vi "ADC Data capture and Process_new.vi"(0 "ADC Output Read Method":T2(ring)=enum."Read .dat file", 1 "Select the Tab to project":T1(ring)=enum."ADC Sine", 2 "ADC Input":enum16{"Sine Wave", "Ramp / Triangle"}(ring), 3 "No.of samples(SNR)":i32=4096, 4 "Resolution":i32=12, 5 "active edge":i32(ring)=10280, 6 "Inputs for Dyanmic para":T9={"Fundamental Frequency"=100000.0, "Sampling Frequncy"=3999610.0, "No of Harmonics"=9, "Window"=enum."7 Term B-Harris", "Blackman (fundamental power) bins)"=1.0}, 7 "Samples per Channel":i32=4096 caption="No.of Samples(capture)", 8 "Oversampling":bool, 9 "Oversampling ratio":i32, 10 "Drop LSB":bool, 11 "Save data":T15, 12 "Waveform":i64[](array[numeric]), 13 "Path to Read":path=path "C/Users/a0230227/Desktop/save.dat", 14 "Start & Stop Bit":cluster{"Start":i32, "Stop":i32}={"Start"=40, "Stop"=4055}, 15 "length":i32=4096, 17 "Set_Freq":dbl=100017.0, 24 "path to save":T14={"Path to Save plot"=path "D/Tenor_176P/DYN_PAR_C004/DAT/D001_TEMPP30C_VDD1.2_VDDA3.3_16B_SE_ADCA__vicA_aggX_PLT_CAP_200821_1740_33.jpg", "Path to Raw Data plot"=path "D/Tenor_176P/DYN_PAR_C004/DAT/D001_TEMPP30C_VDD1.2_VDDA3.3_16B_SE_ADCA__vicA_aggX_RAW_DAT_200821_1740_33.csv"}) -> (18 "Min Max":T4, 19 "detected Throughput":dbl, 20 "output cluster":T7, 21 "Dynamic Parameters":T8, 22 "max code":ext, 23 "min code":ext, 25 "Valid Capture":bool)   [LabVIEW 2019] (continued)
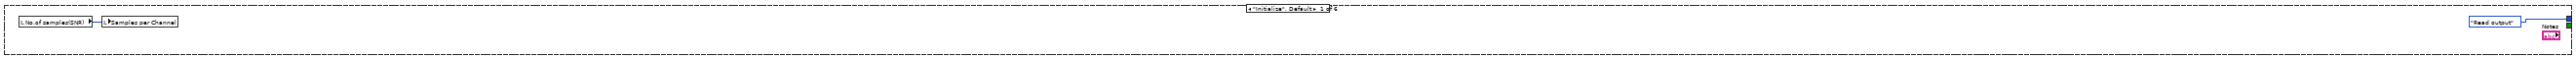
[diagram p2: hidden frame]
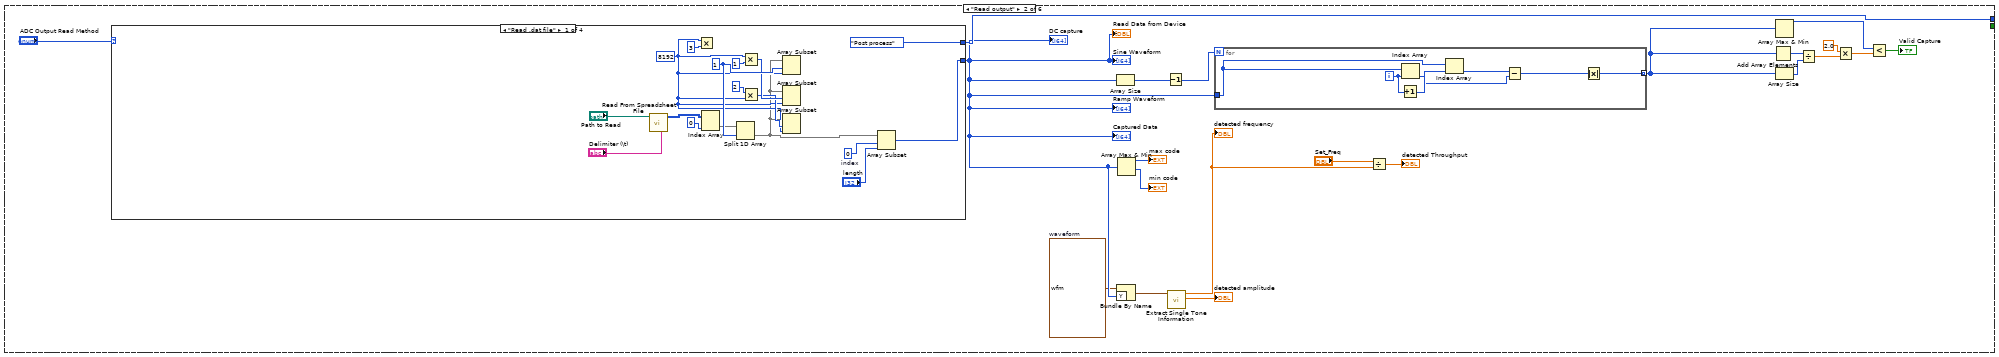
[diagram p3: hidden frame]
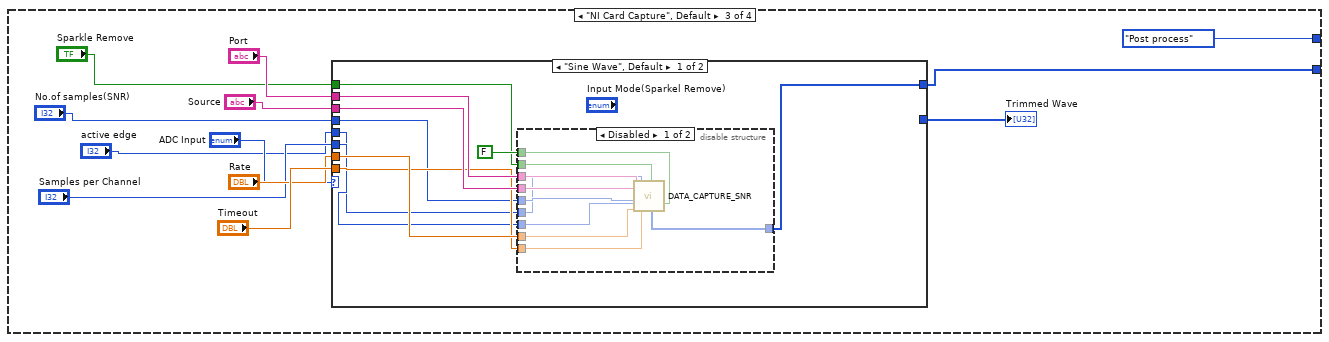
[diagram p5: hidden frame]
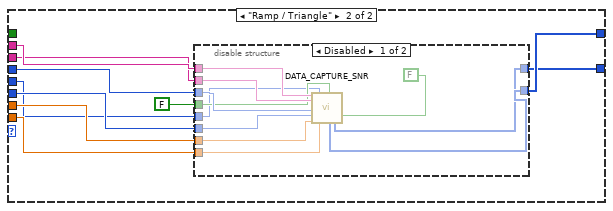
[diagram p7: hidden frame]
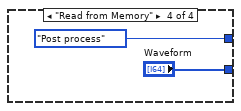
[diagram p9: hidden frame]
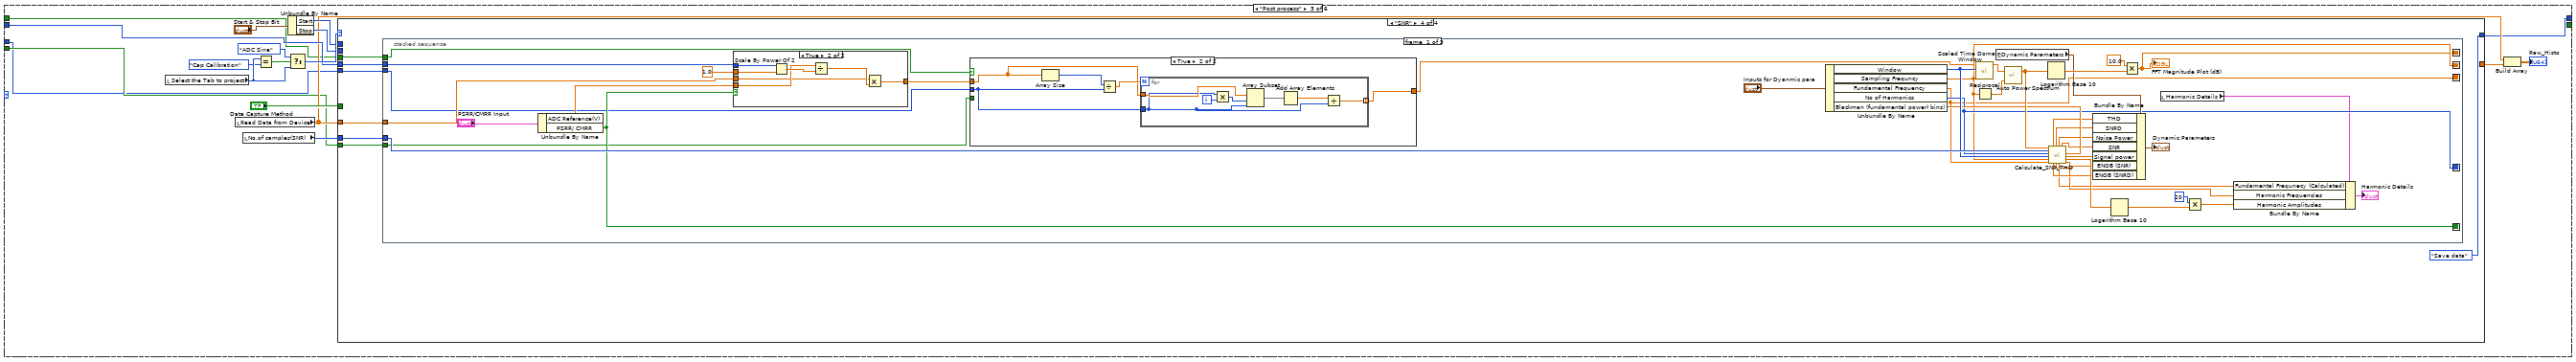
[diagram p10: hidden frame]
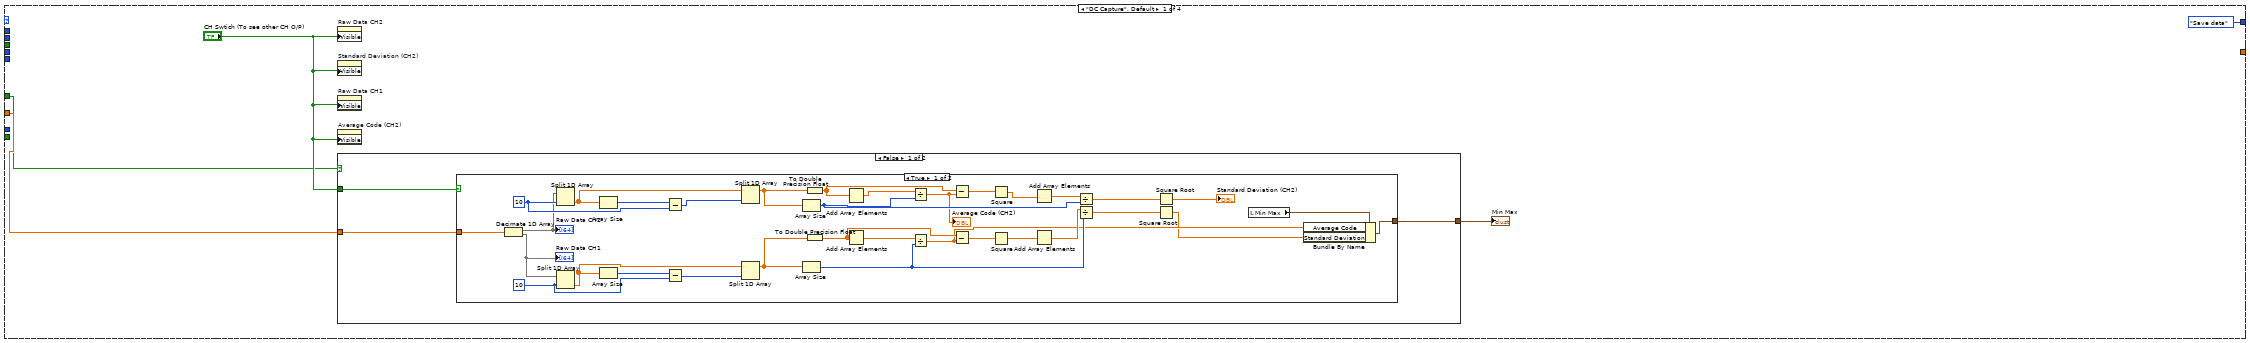
[diagram p11: hidden frame]
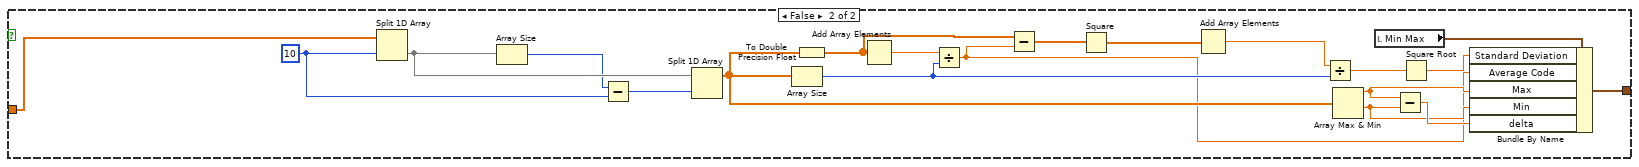
[diagram p12: hidden frame]
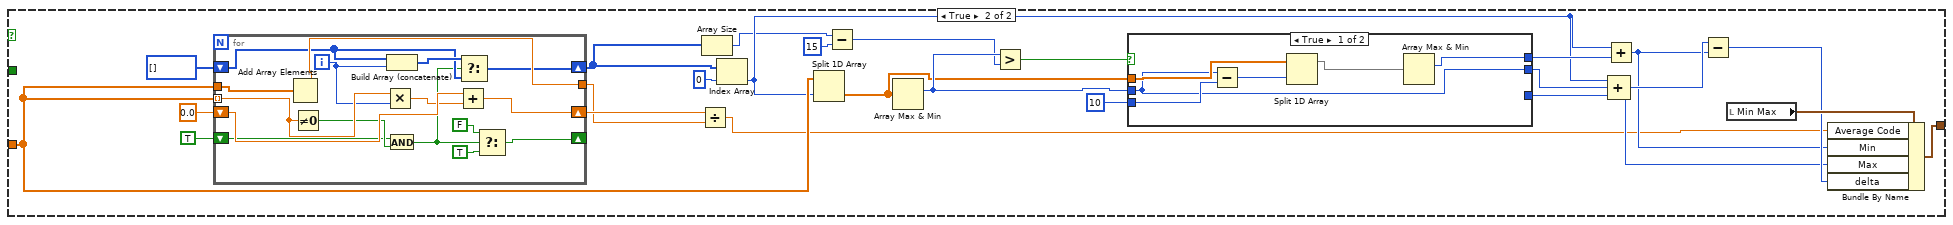
[diagram p13: hidden frame]
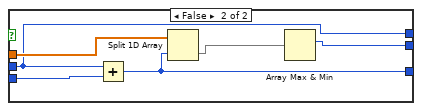
[diagram p14: hidden frame]
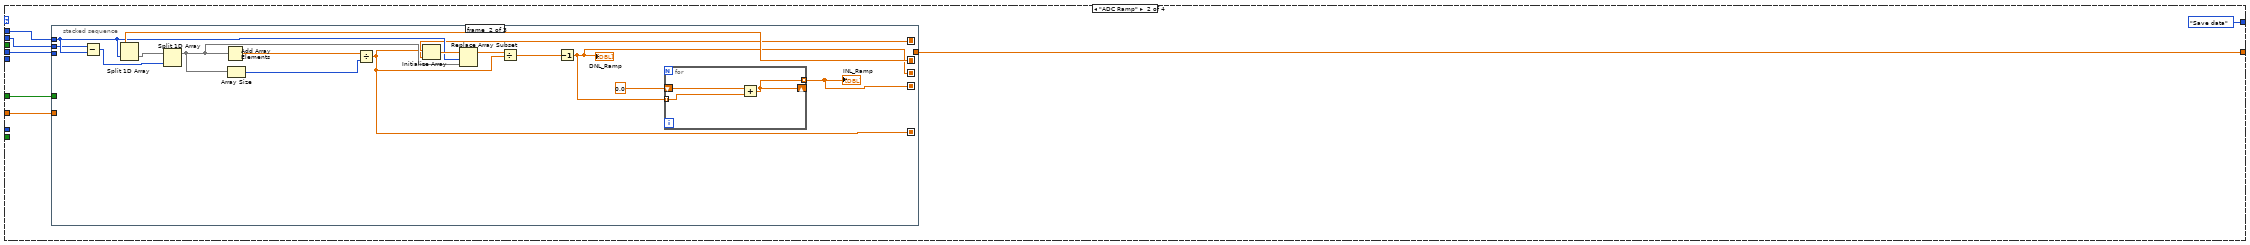
[diagram p15: hidden frame]
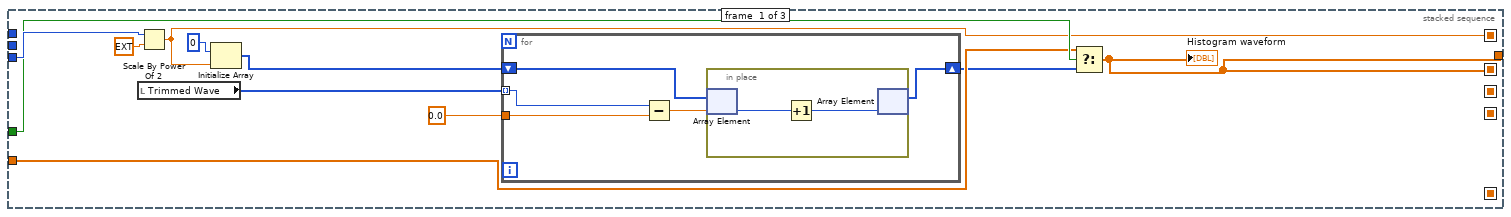
[diagram p16: hidden frame]
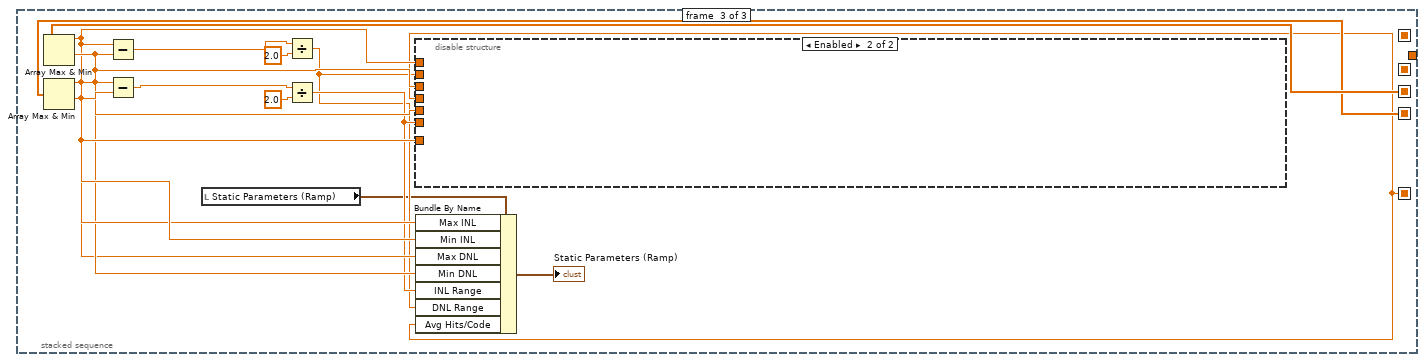
[diagram p17: hidden frame]
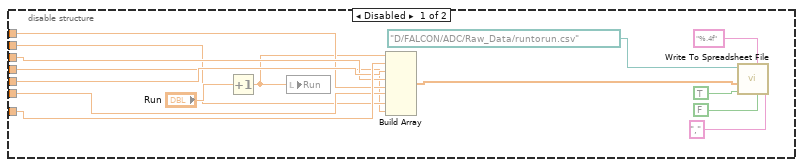
[diagram p18: hidden frame]
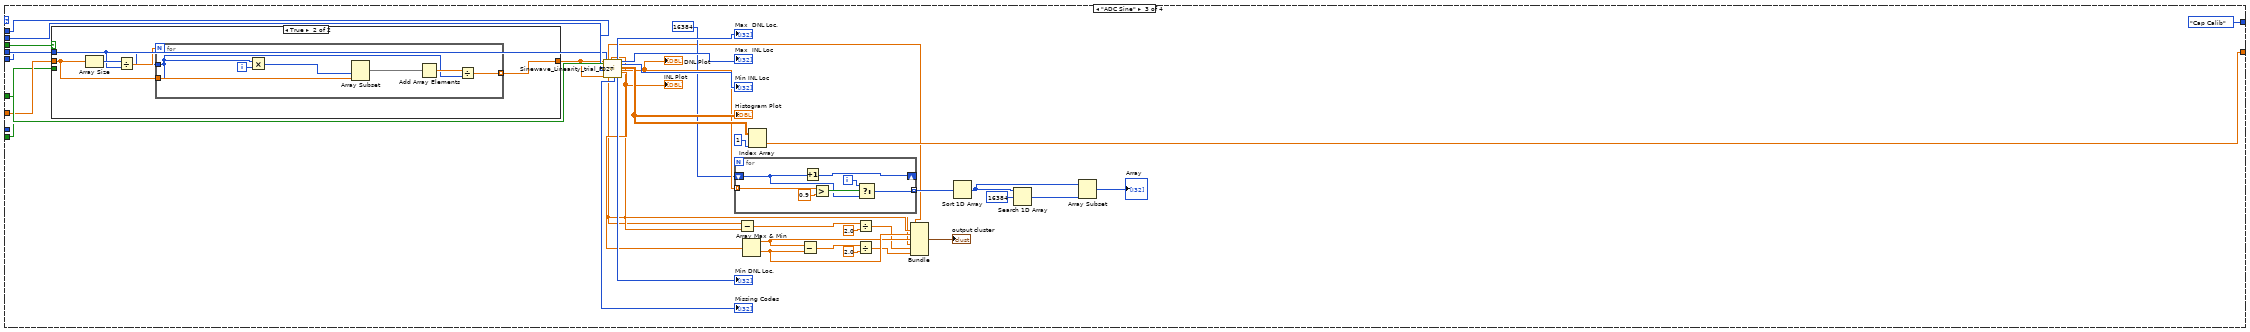
[diagram p19: hidden frame]
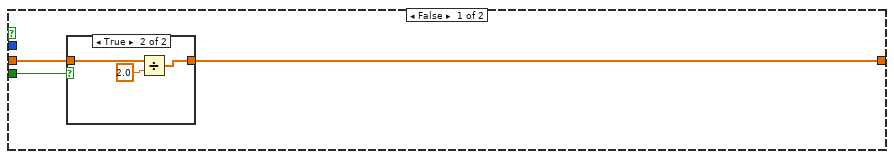
[diagram p20: hidden frame]
                n289 = local read "Histogram waveform"() -> (w742:dbl[])
                n290 = local read "Ramp Waveform"() -> (w743:i64[])
                n291 = local read "DNL_Ramp"() -> (w745:dbl[])
                n292 = local read "INL_Ramp"() -> (w744:dbl[])
                n293 = call-poly <vilib>:"Write Delimited Spreadsheet.vi"("file path (dialog if empty)"=w741, "1D data"=string[] ["ADC Raw data", "DNL", "INL", "Histogram"], "append to file? (new file:F)"=TRUE, "delimiter (\\t)"="" ("delimiter (\\t)")) -> ("new file path (Not A Path if cancelled)"=w737:path)  [unwired: 10 in, 1 out]
                n294 = Build Array(w743, w745, w744, w742) -> (w735:dbl[][])
                n295 = call-poly <vilib>:"Write Delimited Spreadsheet.vi"("file path (dialog if empty)"=w737, "2D data"=w735, "append to file? (new file:F)"=w736, "transpose? (no:F)"=w736) -> ()  [unwired: 10 in, 2 out]
              }
            }
            "Main Tab" <- 3 ("Select Tab")
            "Ramp" <- 2 ("Select Tab")
          }
          frame "ADC Sine", Default {
            n296 = case shown="False" w747 {
              tunnel: w749 -> [_ w752]
              frame False {
              }
              frame True {
                n297 = Current VI's Path() -> (path=w753:path)
                n298 = call "Take fron panel screenshot.vi"("VI path"=w753, "Image path"=w752, "Visible area only? (f)"=FALSE, "File type (.jpg)"=enum16{".bmp", ".png", ".jpg"}.".png") -> ()  [unwired: 4 in, 1 out]
              }
            }
            n299 = case shown="False" w746 {
              tunnel: w750 -> [_ w761]
              frame False {
              }
              frame True {
                w757 = "," ("delimiter (\\t)")
                n300 = local read "Histogram Plot"() -> (w765:dbl[][])
                n301 = local read "Sine Waveform"() -> (w756:i64[])
                n302 = local read "DNL Plot"() -> (w768:dbl[])
                n303 = local read "INL Plot"() -> (w767:dbl[])
                n304 = Index Array(array=w765, index (row)=1 ("disabled index (col)")) -> (element=w764:dbl[])  [unwired: 1 in]
                n305 = call-poly <vilib>:"Write To Spreadsheet File.vi"("delimiter (\\t)"=w757, "1D data"=string[] ["DNL", "INL", "Histogram", "Rawdata"], "file path (dialog if empty)"=w761) -> ("new file path (Not A Path if cancelled)"=w760:path)  [unwired: 5 in]
                n306 = Build Array(w768, w767, w764, w756) -> (w766:dbl[][])
                n307 = call-poly <vilib>:"Write To Spreadsheet File.vi"("delimiter (\\t)"=w757, "transpose? (no:F)"=TRUE, "append to file? (new file:F)"=TRUE, "2D data"=w766, "file path (dialog if empty)"=w760) -> ()  [unwired: 3 in, 1 out]
              }
            }
            n308 = local write "Main Tab"(4) -> ()
            "Sine" <- 1
          }
          frame "SNR" {
            n309 = case shown="True" w770 {
              tunnel: w773 -> [_ w775]
              frame False {
              }
              frame True {
                n310 = Current VI's Path() -> (path=w776:path)
                n311 = call "Take fron panel screenshot.vi"("VI path"=w776, "Image path"=w775, "Visible area only? (f)"=FALSE, "File type (.jpg)"=enum16{".bmp", ".png", ".jpg"}.".png") -> ()  [unwired: 4 in, 1 out]
              }
            }
            n312 = case shown="True" w769 {
              tunnel: w772 -> [_ w783]
              frame False {
              }
              frame True {
                n313 = local read "FFT Plot"() -> (w787:cluster{dbl[], dbl[]})
                n314 = local read "Captured Data"() -> (w786:i64[])
                n315 = Unbundle(w787) -> (w785:dbl[], w784:dbl[])
                n316 = Build Array(w786, w785, w784) -> (w782:dbl[][])
                n317 = call-poly <vilib>:"Write Delimited Spreadsheet.vi"("file path (dialog if empty)"=w783, "2D data"=w782, "append to file? (new file:F)"=TRUE, "transpose? (no:F)"=TRUE, "delimiter (\\t)"="," ("delimiter (\\t)")) -> ()  [unwired: 9 in, 2 out]
              }
            }
            n318 = local write "Main Tab"(5) -> ()
            "SNR" <- 2
          }
          frame "Cap Calibration" {
            n319 = local write "Main Tab"(6) -> ()
          }
          frame "DC Capture" {
            n320 = case shown="True" w789 {
              tunnel: w790 -> [_ w795]
              frame False {
              }
              frame True {
                w793 = TRUE ("transpose? (no:F)")
                n321 = local read "DC capture"() -> (w794:i64[])
                n322 = call-poly <vilib>:"Write Delimited Spreadsheet.vi"("file path (dialog if empty)"=w795, "1D data"=w794, "append to file? (new file:F)"=w793, "transpose? (no:F)"=w793, "delimiter (\\t)"="" ("delimiter (\\t)")) -> ()  [unwired: 9 in, 2 out]
              }
            }
            n323 = local write "Main Tab"(2) -> ()
          }
        }
      }
      frame "Exit" {
        n324 = disable-structure shown="Enabled" {
          frame Enabled {
            w797 = FALSE ("Save INL/DNL Plot(Ramp)")
            n325 = local read "Save data"() -> (w799:T15)
            n326 = Bundle By Name(cluster=w799, "Save INL/DNL Plot(Ramp)"=w797, "Save SNR Plot"=w797, "Save INL/DNL Plot(Sine)"=w797, "Save INL/DNL Raw Data(Ramp)"=w797, "Save SNR Raw Data"=w797, "Save INL/DNL Raw Data(Sine)"=w797, "Save  Raw Data(Sine)"=w797) -> (w798:T15)
            n327 = local write "Save data"(w798) -> ()
          }
          frame Disabled {
          }
        }
        n328 = disable-structure shown="Enabled" {
          frame Disabled {
            n329 = local write item#-1(u32 12000 ("Wait time to Read Memory \n(To complete Conv) mS")) -> ()
          }
          frame Enabled {
          }
        }
      }
    }
  }
